vi "MeasureInfoToUserInput.vi"(11 "MeasureInfo":T1 {"MeasStopInfo"."flags" format="x%x"}) -> (1 "adc_resolution_digital":i32, 2 "ADC Resolution Bits":T11=12 items=["-1"=255, "1"=0, "4"=2, "16"=4, "64"=6, "256"=8, "1024"=10, "4096"=12], 3 "User Input":T12={"tac_range"=50.0, "tac_gain"=3, "tac_offset"=12.0, "tac_limit_high"=96.0, "tac_limit_low"=3.0, "collect_time"=2.0, "sync_threshold"=-71.0, "sync_zc_level"=-5.0, "sync_freq_div"=1, "cfd_limit_low"=-50.0, "cfd_zc_level"=9.8} {"sync_freq_div" items=["1"=1, "2"=2, "4"=4]; "cfd_zc_level" min=-96 max=96 step=0.1 format="%#_3g"; "cfd_limit_low" min=-500 max=0 step=0.1 format="%#_3g"; "sync_zc_level" min=-96 max=96 step=0.1 format="%#_3g"; "sync_threshold" min=-500 max=-20 step=0.1 format="%#_3g"; "tac_limit_low" format="%.3g"; "tac_limit_high" min=0 max=100 step=0.1 format="%.3g"; "collect_time" min=1e-07 max=100000 step=0.001; "tac_offset" min=0 max=100 step=0.1 format="%.4g"; "tac_gain" min=1 max=15 step=1; "tac_range" format="%^#_6g"})   [LabVIEW 2017]
doc: "This VI demonstrates how specific parameters can be entered into an ASCII SetUp-block replacing their default values.\nProvide the Key up to and including the format specifier and trailing comma.\n\ninfo@becker-hickl.com"
uses:
  Example_Controls/UserInput.ctl
  SPC_Wrappers/SPC_Controls/ADCResolution.ctl
  SPC_Wrappers/SPC_Controls/MeasureInfo.ctl
  SPC_Wrappers/SPC_Controls/MeasureInfo_PartB.ctl
  SPC_Wrappers/SPC_Controls/MeasStopInfo.ctl
  SPC_Wrappers/SPC_Controls/MeasFCSInfo.ctl
  SPC_Wrappers/SPC_Controls/MeasureInfo_PartE.ctl
  SPC_Wrappers/SPC_Controls/MeasHISTInfo.ctl
  SPC_Wrappers/SPC_Controls/HISTInfoExt.ctl
  SPC_Wrappers/SPC_Controls/MeasureInfo_PartI.ctl
  SPC_Wrappers/SPC_Controls/MeasureInfo_PartK.ctl
  SPC_Wrappers/SPC_Controls/MeasureInfo_PartM.ctl
panel:
  # "TAC / Time Range"
  # "CFD"
  # "(start)"
  # "SYNC"
  # "(stop)"
  # "range"
  # "gain"
  # "threshold(LL)"
  # "offset"
  # "limit high"
  # "limit low"
  # "zero cross(ZC)"
  # "Collection Time"
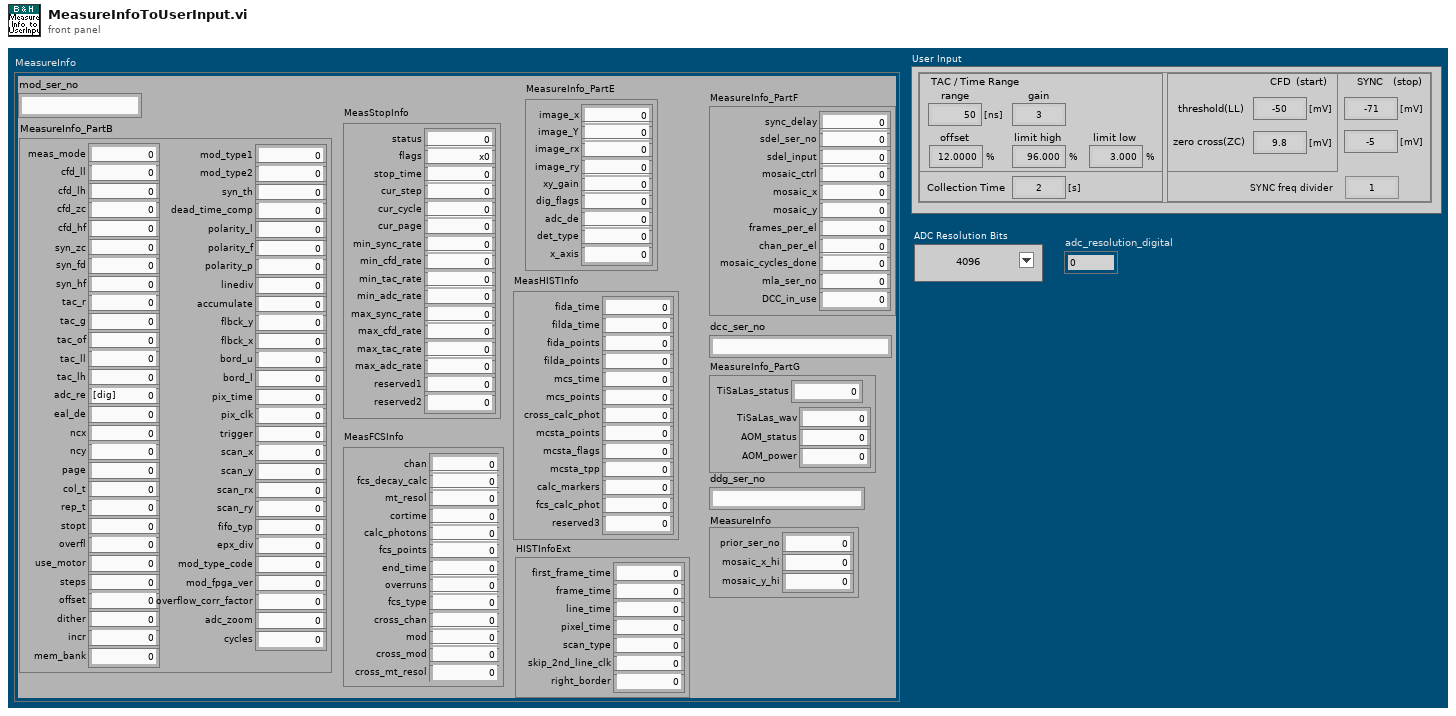
[diagram p1: front panel]
types:
  T1 = typedef "MeasureInfo.ctl" = cluster{"mod_ser_no":string, "MeasureInfo_PartB":T2, "MeasStopInfo":T3, "MeasFCSInfo":T4, "MeasureInfo_PartE":T5, "MeasHISTInfo":T6, "HISTInfoExt":T7, "MeasureInfo_PartF":T8, "dcc_ser_no":string, "MeasureInfo_PartG":T9, "ddg_ser_no":string, "MeasureInfo":T10}
  T2 = typedef "MeasureInfo_PartB.ctl" = cluster{"meas_mode":i16, "cfd_ll":sgl, "cfd_lh":sgl, "cfd_zc":sgl, "cfd_hf":sgl, "syn_zc":sgl, "syn_fd":i16, "syn_hf":sgl, "tac_r":sgl, "tac_g":i16, "tac_of":sgl, "tac_ll":sgl, "tac_lh":sgl, "adc_re":i16, "eal_de":i16, "ncx":i16, "ncy":i16, "page":u16, "col_t":sgl, "rep_t":sgl, "stopt":i16, "overfl":i8, "use_motor":i16, "steps":u16, "offset":sgl, "dither":i16, "incr":i16, "mem_bank":i16, "mod_type1":u64, "mod_type2":u64, "syn_th":sgl, "dead_time_comp":i16, "polarity_l":i16, "polarity_f":i16, "polarity_p":i16, "linediv":i16, "accumulate":i16, "flbck_y":i32, "flbck_x":i32, "bord_u":i32, "bord_l":i32, "pix_time":sgl, "pix_clk":i16, "trigger":i16, "scan_x":i32, "scan_y":i32, "scan_rx":i32, "scan_ry":i32, "fifo_typ":i16, "epx_div":i32, "mod_type_code":u16, "mod_fpga_ver":u16, "overflow_corr_factor":sgl, "adc_zoom":i32, "cycles":i32}
  T3 = typedef "MeasStopInfo.ctl" = cluster{"status":u16, "flags":u16, "stop_time":sgl, "cur_step":i32, "cur_cycle":i32, "cur_page":i32, "min_sync_rate":sgl, "min_cfd_rate":sgl, "min_tac_rate":sgl, "min_adc_rate":sgl, "max_sync_rate":sgl, "max_cfd_rate":sgl, "max_tac_rate":sgl, "max_adc_rate":sgl, "reserved1":i32, "reserved2":sgl}
  T4 = typedef "MeasFCSInfo.ctl" = cluster{"chan":u16, "fcs_decay_calc":u16, "mt_resol":u32, "cortime":sgl, "calc_photons":u32, "fcs_points":i32, "end_time":sgl, "overruns":u16, "fcs_type":u16, "cross_chan":u16, "mod":u16, "cross_mod":u16, "cross_mt_resol":u32}
  T5 = typedef "MeasureInfo_PartE.ctl" = cluster{"image_x":i32, "image_Y":i32, "image_rx":i32, "image_ry":i32, "xy_gain":i16, "dig_flags":i16, "adc_de":i16, "det_type":i16, "x_axis":i16}
  T6 = typedef "MeasHISTInfo.ctl" = cluster{"fida_time":sgl, "filda_time":sgl, "fida_points":i32, "filda_points":i32, "mcs_time":sgl, "mcs_points":i32, "cross_calc_phot":u32, "mcsta_points":u16, "mcsta_flags":u16, "mcsta_tpp":u32, "calc_markers":u32, "fcs_calc_phot":u32, "reserved3":u32}
  T7 = typedef "HISTInfoExt.ctl" = cluster{"first_frame_time":sgl, "frame_time":sgl, "line_time":sgl, "pixel_time":sgl, "scan_type":i16, "skip_2nd_line_clk":i16, "right_border":u32}
  T8 = typedef "MeasureInfo_PartI.ctl" = cluster{"sync_delay":sgl, "sdel_ser_no":u16, "sdel_input":i8, "mosaic_ctrl":i8, "mosaic_x":u8, "mosaic_y":u8, "frames_per_el":i16, "chan_per_el":i16, "mosaic_cycles_done":i32, "mla_ser_no":u16, "DCC_in_use":u8}
  T9 = typedef "MeasureInfo_PartK.ctl" = cluster{"TiSaLas_status":u16, "TiSaLas_wav":u16, "AOM_status":u8, "AOM_power":u8}
  T10 = typedef "MeasureInfo_PartM.ctl" = cluster{"prior_ser_no":i32, "mosaic_x_hi":u8, "mosaic_y_hi":u8}
  T11 = typedef "ADCResolution.ctl" = i16
  T12 = typedef "UserInput.ctl" = cluster{"tac_range":sgl, "tac_gain":i16, "tac_offset":sgl, "tac_limit_high":sgl, "tac_limit_low":sgl, "collect_time":sgl, "sync_threshold":sgl, "sync_zc_level":sgl, "sync_freq_div":i16, "cfd_limit_low":sgl, "cfd_zc_level":sgl}
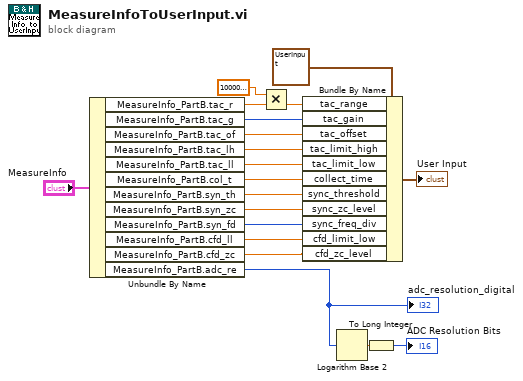
[diagram p0: block diagram]
diagram:
  n1 = Unbundle By Name("MeasureInfo") -> ("MeasureInfo_PartB.tac_r"=w14:sgl, "MeasureInfo_PartB.tac_g"=w11:i16, "MeasureInfo_PartB.tac_of"=w10:sgl, "MeasureInfo_PartB.tac_lh"=w9:sgl, "MeasureInfo_PartB.tac_ll"=w8:sgl, "MeasureInfo_PartB.col_t"=w7:sgl, "MeasureInfo_PartB.syn_th"=w6:sgl, "MeasureInfo_PartB.syn_zc"=w5:sgl, "MeasureInfo_PartB.syn_fd"=w4:i16, "MeasureInfo_PartB.cfd_ll"=w3:sgl, "MeasureInfo_PartB.cfd_zc"=w2:sgl, "MeasureInfo_PartB.adc_re"=w16:i16)
  "adc_resolution_digital" <- w16
  n2 = Multiply(x=sgl 1000000000.0, y=w14) -> (x*y=w13:sgl)
  n3 = Bundle By Name(cluster=T12 {"tac_range"=50.0, "tac_gain"=3, "tac_offset"=12.0, "tac_limit_high"=96.0, "tac_limit_low"=3.0, "collect_time"=2.0, "sync_threshold"=-71.0, "sync_zc_level"=-5.0, "sync_freq_div"=1, "cfd_limit_low"=-50.0, "cfd_zc_level"=9.8} ("User Input"), "tac_range"=w13, "tac_gain"=w11, "tac_offset"=w10, "tac_limit_high"=w9, "tac_limit_low"=w8, "collect_time"=w7, "sync_threshold"=w6, "sync_zc_level"=w5, "sync_freq_div"=w4, "cfd_limit_low"=w3, "cfd_zc_level"=w2) -> (→"User Input":T12)
  n4 = Logarithm Base 2(1:w16) -> (0:w19:dbl)
  n5 = To Long Integer(number=w19) -> (32bit integer=→"ADC Resolution Bits":i32)
